vi "String and values cluster array to individual array.vi"(0 "Strings and Values In":T1) -> (1 "String Array Out":string[](array[string]), 2 "Value Array Out":i32[](array[numeric]))   [LabVIEW 2020, in "Field Interfaces.lvlib"]
uses:
  <vilib>/Utility/miscctls.llb/LVStringsAndValuesArrayTypeDef.ctl
  Field Interfaces.lvlib
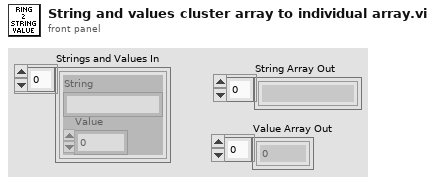
[diagram p1: front panel]
types:
  T1 = typedef "LVStringsAndValuesArrayTypeDef.ctl" = cluster{"String":string, "Value":ext}[]
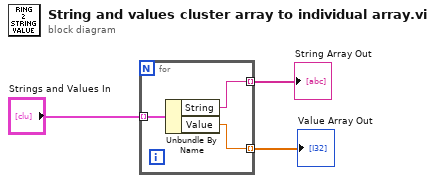
[diagram p0: block diagram]
diagram:
  n1 = for {
    tunnel: "Strings and Values In" -> [w6] mode=indexing
    tunnel: [w5] -> w2 mode=indexing
    tunnel: [w4] -> w1 mode=indexing
    n2 = Unbundle By Name(w6) -> ("String"=w5:string, "Value"=w4:ext)
  }
  "String Array Out" <- w2
  "Value Array Out" <- w1
